vi "Remove View from Subpanel.vi"(0 "GUI Container Actor in":refnum<class "GUI Container Actor.lvclass">, 9 "Subpanel":string, 11 "error in (no error)":errorcluster) -> (4 "GUI Container Actor out":refnum<class "GUI Container Actor.lvclass">, 15 "error out":errorcluster)   [LabVIEW 2017, in "GUI Views.lvlib" / "GUI Container Actor.lvclass"]
doc: "Removes the Front Panel of a specified Actor Core VI of the the specified View class hierarchy from a specified subpanel\n\n<b> View </b> String theat contains the name of the View\n\n<b> View Hierarchy Level</b> the level on the subclassing hierarchy of the GUI View actor, it is used to choose the Actor Core Front Panel among all the exisiting sublcasses of the GUI VIew Actor present in the View specified above\n\n<b>Subpanel</b> string designating in which subpanel the Front Panel specified in the above terminals has to be inserted"
uses:
  GUI Container Actor.lvclass
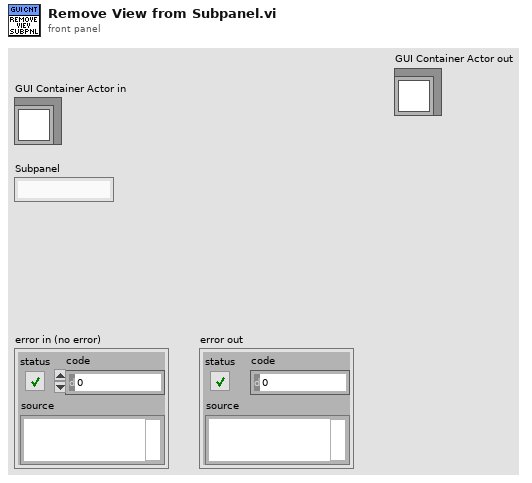
[diagram p1: front panel]
types:
  T1 = typedef "GUI Views.lvlib/GUI Container Actor.lvclass/Subpanel Status.ctl" = cluster{"Subpanel Ref":refnum<vi>, "Inserted View":string, "Inserted View Hierarchy Level":i32}
  T2 = typedef "GUI Views.lvlib/GUI Container Actor.lvclass/View Status.ctl" = cluster{"View Details":T3, "Front Panel Statuses":T4[]}
  T3 = typedef "GUI Views.lvlib/GUI Container Actor.lvclass/View Details.ctl" = cluster{"Enqueuer":refnum<class "Message Enqueuer.lvclass">, "VI References":refnum<vi>[], "FP References":refnum<vi>[]}
  T4 = typedef "GUI Views.lvlib/GUI Container Actor.lvclass/FP Status.ctl" = cluster{"FP Open":bool, "Inserted in Subpanel":bool, "Subpanel":string}
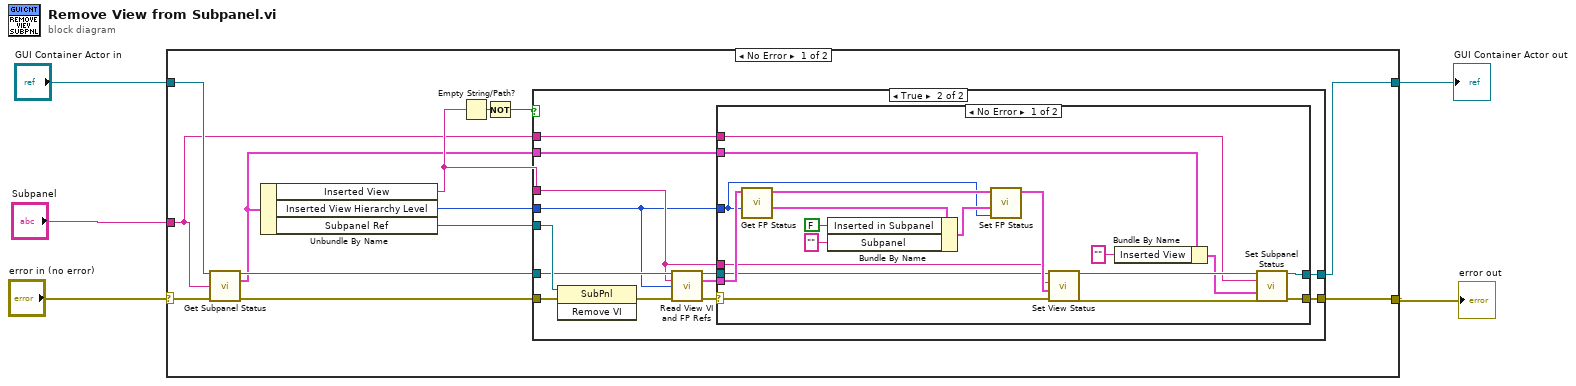
[diagram p0: block diagram]
diagram:
  n1 = case shown="No Error" "error in (no error)" {
    selector: "error in (no error)" -> [w17 w55]
    tunnel: [w18 w55] -> w5
    tunnel: "GUI Container Actor in" -> [w15 w56]
    tunnel: "Subpanel" -> [w7 _]
    tunnel: [w8 w56] -> w1
    frame No Error {
      n2 = call "Get Subpanel Status.vi"("GUI Container Actor in"=w15, "Subpanel"=w7, "error in (no error)"=w17) -> ("GUI Container Actor out"=w11:refnum<class "GUI Container Actor.lvclass">, "Subpanel Status"=w6:T1, "error out"=w16:errorcluster)  [unwired: 9 in, 1 out]
      n3 = Unbundle By Name(w6) -> ("Inserted View"=w9:string, "Inserted View Hierarchy Level"=w10:i32, "Subpanel Ref"=w14:refnum<vi>)
      n4 = Empty String/Path?(string/path=w9) -> (empty?=w13:bool)
      n5 = Not(x=w13) -> (.not. x?=w12:bool)
      n6 = case shown="True" w12 {
        tunnel: [w20 w27] -> w18
        tunnel: w16 -> [w20 w33]
        tunnel: w14 -> [_ w32]
        tunnel: w11 -> [w19 w31]
        tunnel: w10 -> [_ w24]
        tunnel: w9 -> [_ w25]
        tunnel: [w19 w23] -> w8
        tunnel: w7 -> [_ w22]
        tunnel: w6 -> [_ w21]
        frame False {
        }
        frame True {
          n7 = invoke class="SubPnl" method="Remove VI"(reference=w32, error in=w33) -> (error out=w30:errorcluster)  [unwired: 1 in, 2 out]
          n8 = call "Read View VI and FP Refs.vi"("GUI Container Actor in"=w31, "View"=w25, "View Hierarchy Level"=w24, "error in (no error)"=w30) -> ("GUI Container Actor out"=w26:refnum<class "GUI Container Actor.lvclass">, "View Status"=w29:T2, "error out"=w28:errorcluster)  [unwired: 7 in, 2 out]
          n9 = case shown="No Error" w28 {
            selector: w28 -> [w47 w54]
            tunnel: w29 -> [w51 _]
            tunnel: [w40 w54] -> w27
            tunnel: w26 -> [w45 w53]
            tunnel: w25 -> [w44 _]
            tunnel: w24 -> [w42 _]
            tunnel: [w39 w53] -> w23
            tunnel: w22 -> [w37 _]
            tunnel: w21 -> [w36 _]
            frame No Error {
              n10 = call "Get FP Status.vi"("View Hierarchy Level"=w42, "View Status in"=w51) -> ("FP Status"=w43:T4, "View Status out"=w52:T2)  [unwired: 8 in]
              n11 = Bundle By Name(cluster=w43, "Inserted in Subpanel"=FALSE, "Subpanel"="") -> (w48:T4)
              n12 = call "Set FP Status.vi"("View Hierarchy Level"=w42, "FP Status"=w48, "View Status in"=w52) -> ("View Status out"=w46:T2)  [unwired: 8 in]
              n13 = call "Set View Status.vi"("error in (no error)"=w47, "View Status"=w46, "View"=w44, "GUI Container Actor in"=w45) -> ("error out"=w41:errorcluster, "GUI Container Actor out"=w38:refnum<class "GUI Container Actor.lvclass">)  [unwired: 5 in, 1 out]
              n14 = Bundle By Name(cluster=w36, "Inserted View"="") -> (w34:T1)
              n15 = call "Set Subpanel Status.vi"("GUI Container Actor in"=w38, "Subpanel"=w37, "Subpanel Status"=w34, "error in (no error)"=w41) -> ("GUI Container Actor out"=w39:refnum<class "GUI Container Actor.lvclass">, "error out"=w40:errorcluster)  [unwired: 9 in, 1 out]
            }
            frame Error {
            }
          }
        }
      }
    }
    frame Error {
    }
  }
  "error out" <- w5
  "GUI Container Actor out" <- w1
